vi "LVPortUpdateObjectMapDataValueToComplexNumberOrArrayVariant.vi"(0 "UpdatedData":cdb[](array[numeric]), 5 "Sizes":i32[](array[numeric]), 7 "UpdateAt":i32[](array[numeric]), 9 "Has Value":bool, 11 "SourceValue":variant) -> (4 "Value":variant, 8 "Invalid Indexing or errored value":bool)   [LabVIEW 2017]
uses:
  <vilib>/Utility/Data Type/Type Definitions/Data Type.ctl
  <vilib>/Utility/Data Type/NI_Data Type.lvlib
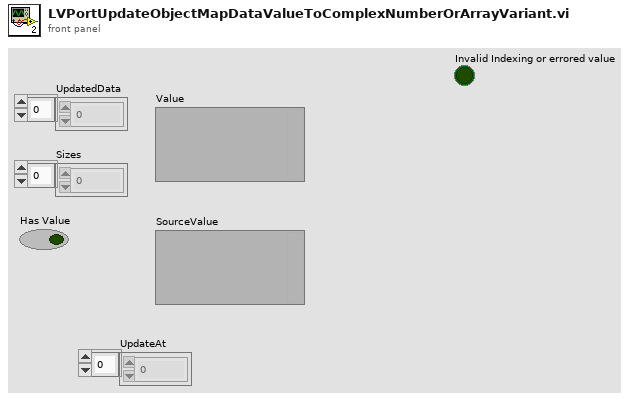
[diagram p1: front panel]
types:
  T1 = typedef "NI_Data Type.lvlib/Data Type.ctl" = enum8{"Invalid Type", "Void", "I8", "I16", "I32", "I64", "U8", "U16", "U32", "U64", "Single Float", "Double Float", "Extended Float", "Single Complex", "Double Complex", "Extended Complex", "Enum U8", "Enum U16", "Enum U32", "Enum U64", "Single Float With Unit", "Double Float With Unit", "Extended Float With Unit", "Single Complex with Unit", "Double Complex with Unit", "Extended Complex with Unit", "Boolean", "String", "Path", "Picture", "Tag", "Array", "Cluster", "Variant", "LV Variant", "Waveform", "Timestamp", "Digital Waveform", "Digital Data", "ExpressData", "Refnum", "External Data", "VI", "Poly VI", "LabVIEW Class Instance", "Fixed Point"}
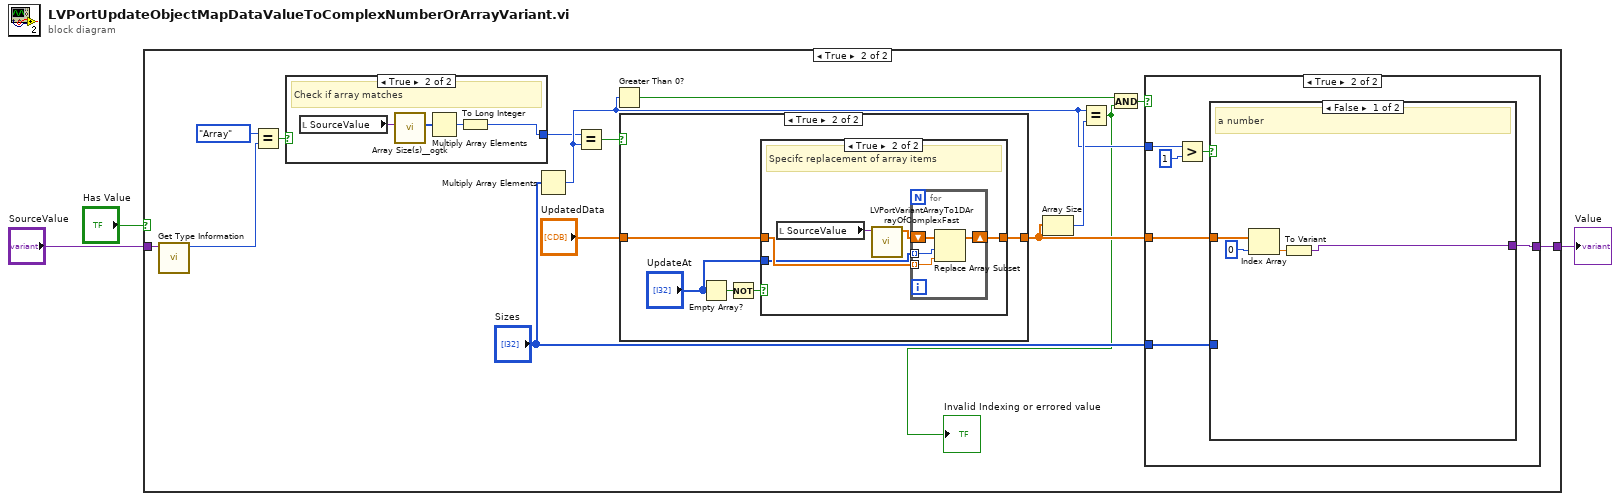
[diagram p0: block diagram]
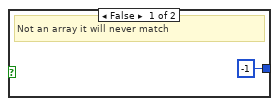
[diagram p3: hidden frame]
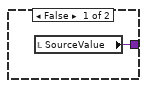
[diagram p6: hidden frame]
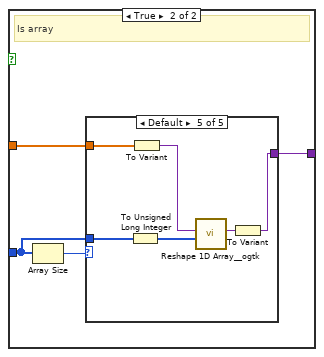
[diagram p7: hidden frame]
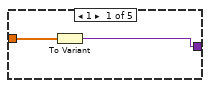
[diagram p8: hidden frame]
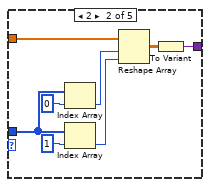
[diagram p9: hidden frame]
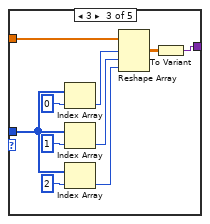
[diagram p10: hidden frame]
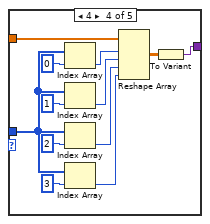
[diagram p11: hidden frame]
diagram:
  n1 = case shown="True" "Has Value" {
    tunnel: [w4 w14] -> w2
    tunnel: "SourceValue" -> [w4 w11]
    frame False {
    }
    frame True {
      n2 = call <vilib>:"Get Type Information.vi"("Variant"=w11) -> ("Type"=w13:T1)  [unwired: 6 in, 4 out]
      n3 = Equal?(x=Data_Type."Array" ("Type"), y=w13) -> (x = y?=w6:bool)
      n4 = case shown="True" w6 {
        tunnel: [-1 w22] -> w7
        frame False {
          # "Not an array it will never match"
        }
        frame True {
          # "Check if array matches"
          n5 = local read "SourceValue"() -> (w21:variant)
          n6 = call <userlib>:"Array Size(s)__ogtk.vi"("Array"=w21) -> ("Size(s)"=w23:u32[])  [unwired: 8 in, 2 out]
          n7 = Multiply Array Elements(1:w23) -> (0:w24:u32)
          n8 = To Long Integer(number=w24) -> (32bit integer=w22:i32)
        }
      }
      n9 = Multiply Array Elements(1:"Sizes") -> (0:w10:i32)
      n10 = Equal?(x=w7, y=w10) -> (x = y?=w9:bool)
      n11 = Greater Than 0?(x=w10) -> (x > 0?=w15:bool)
      n12 = case shown="True" w9 {
        tunnel: [w25 w28] -> w17
        tunnel: "UpdatedData" -> [w25 w26]
        frame False {
        }
        frame True {
          n13 = Empty Array?(array="UpdateAt") -> (empty?=w30:bool)
          n14 = Not(x=w30) -> (.not. x?=w29:bool)
          n15 = case shown="True" w29 {
            tunnel: w26 -> [w31 w35]
            tunnel: [w31 w33] -> w28
            tunnel: "UpdateAt" -> [_ w34]
            frame False {
              # "The new array is the new value"
            }
            frame True {
              # "Specifc replacement of array items"
              n16 = local read "SourceValue"() -> (w32:variant)
              n17 = call "LVPortVariantArrayTo1DArrayOfComplexFast.vi"("Variant Real Array"=w32) -> ("1D Array"=w36:cdb[])  [unwired: 8 in, 2 out]
              n18 = for {
                shift-right: [w37] -> w33
                shift-left: w36 -> [w40]
                tunnel: w35 -> [w39] mode=indexing
                tunnel: w34 -> [w38] mode=indexing
                n19 = Replace Array Subset(array=w40, new element=w39, index=w38) -> (w37:cdb[])
              }
            }
          }
        }
      }
      n20 = Array Size(array=w17) -> (size(s)=w16:i32)
      n21 = Equal?(x=w10, y=w16) -> (x = y?=w5:bool)
      "Invalid Indexing or errored value" <- w5
      n22 = And(x=w15, y=w5) -> (x .and. y?=w18:bool)
      n23 = case shown="True" w18 {
        tunnel: "Sizes" -> [_ w44]
        tunnel: w17 -> [_ w45]
        tunnel: [w41 w43] -> w14
        tunnel: w10 -> [_ w47]
        frame False {
          n24 = local read "SourceValue"() -> (w41:variant)
        }
        frame True {
          n25 = Greater?(x=w47, y=1) -> (0:w46:bool)
          n26 = case shown="False" w46 {
            tunnel: w45 -> [w51 w53]
            tunnel: w44 -> [_ w52]
            tunnel: [w48 w54] -> w43
            frame False {
              # "a number"
              n27 = Index Array(array=w51, index=0) -> (element=w49:cdb)
              n28 = To Variant(anything=w49) -> (Variant=w48:variant)
            }
            frame True {
              # "Is array"
              n29 = Array Size(array=w52) -> (size(s)=w55:i32)
              n30 = case shown="Default" w55 {
                tunnel: [w56 w58 w66 w76 w92] -> w54
                tunnel: w53 -> [w57 w65 w71 w81 w88]
                tunnel: w52 -> [_ w64 w69 w79 w91]
                frame 1 {
                  n31 = To Variant(anything=w57) -> (Variant=w56:variant)
                }
                frame 2 {
                  n32 = Index Array(array=w64, index=0) -> (element=w63:i32)
                  n33 = Index Array(array=w64, index=1) -> (element=w62:i32)
                  n34 = Reshape Array(w65, w63, w62) -> (w59:cdb[][])
                  n35 = To Variant(anything=w59) -> (Variant=w58:variant)
                }
                frame 3 {
                  n36 = Index Array(array=w69, index=0) -> (element=w75:i32)
                  n37 = Index Array(array=w69, index=1) -> (element=w74:i32)
                  n38 = Index Array(array=w69, index=2) -> (element=w68:i32)
                  n39 = Reshape Array(w71, w75, w74, w68) -> (w67:cdb[][][])
                  n40 = To Variant(anything=w67) -> (Variant=w66:variant)
                }
                frame 4 {
                  n41 = Index Array(array=w79, index=0) -> (element=w87:i32)
                  n42 = Index Array(array=w79, index=1) -> (element=w86:i32)
                  n43 = Index Array(array=w79, index=2) -> (element=w82:i32)
                  n44 = Index Array(array=w79, index=3) -> (element=w78:i32)
                  n45 = Reshape Array(w81, w87, w86, w82, w78) -> (w77:cdb[][][][])
                  n46 = To Variant(anything=w77) -> (Variant=w76:variant)
                }
                frame Default {
                  n47 = To Unsigned Long Integer(number=w91) -> (unsigned 32bit integer=w90:u32[])
                  n48 = To Variant(anything=w88) -> (Variant=w89:variant)
                  n49 = call <userlib>:"Reshape 1D Array__ogtk.vi"("Size(s)"=w90, "1D Array"=w89) -> ("Reshaped VArray"=w93:variant)  [unwired: 8 in, 1 out]
                  n50 = To Variant(anything=w93) -> (Variant=w92:variant)
                }
              }
            }
          }
        }
      }
    }
  }
  "Value" <- w2
